vi "XIPIN_7_Series_FPGAs_Transceivers_Wizard_3_6.vi"   [LabVIEW 2017]
doc: "Use the 7 Series FPGAs Transceivers Wizard to configure one or more Virtex-7/Kintex-7/Artix-7/Zynq FPGA transceivers. Start from scratch, or use an industry standard template. The Wizard generates a custom wrapper for the tranceivers you've selected. In addition, it produces an example design, testbench, and scripts to observe the transceivers operating under simulation and in hardware.\n------------------------------------\n<b>Need License</b> : No"
uses:
  <vilib>/rvi/XilinxIP/XIPIN_XNode/niFpgaXIPIN.xnode
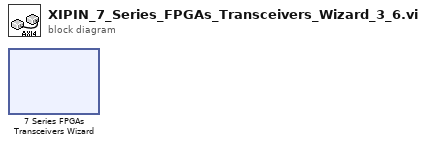
[diagram p0: block diagram]
diagram:
  n1 = xnode ("7 Series FPGAs Transceivers Wizard")() -> ()
